vi "PicoScope4000aAdvancedTriggerSettings.vi"(0 "handle in":i16=16384, 5 "error in":errorcluster, 6 "Trigger Conditions":T4={"Channel A"=1, "Channel B"=0, "Channel C"=0, "Channel D"=0, "Channel E"=0, "Channel F"=0, "Channel G"=0, "Channel H"=0, "Ext"=0, "Aux"=0, "PWQ"=0, "Condition Logic"=0} {"Channel H" items=["Don't Care", "True", "False"]; "Channel G" items=["Don't Care", "True", "False"]; "Channel F" items=["Don't Care", "True", "False"]; "Channel E" items=["Don't Care", "True", "False"]; "PWQ" items=["Don't Care", "True", "False"]; "Aux" items=["Don't Care", "True", "False"]; "Ext" items=["Don't Care", "True", "False"]; "Channel D" items=["Don't Care", "True", "False"]; "Channel C" items=["Don't Care", "True", "False"]; "Channel B" items=["Don't Care", "True", "False"]; "Channel A" items=["Don't Care", "True", "False"]; "Condition Logic" items=["AND", "OR", "XOR"]}, 8 "Channel Trigger Properties":T2={"Channel A Trigger Properties"={"thresholdUpper"=0, "thresholdUpperHysteresis"=0, "thresholdLower"=0, "thresholdLowerHysteresis"=0, "Threshold Mode"=0, "Direction"=2, "Available"=TRUE}, "Channel B Trigger Properties"={"thresholdUpper"=0, "thresholdUpperHysteresis"=0, "thresholdLower"=0, "thresholdLowerHysteresis"=0, "Threshold Mode"=0, "Direction"=2, "Available"=FALSE}, "Channel C Trigger Properties"={"thresholdUpper"=0, "thresholdUpperHysteresis"=0, "thresholdLower"=0, "thresholdLowerHysteresis"=0, "Threshold Mode"=0, "Direction"=2, "Available"=FALSE}, "Channel D Trigger Properties"={"thresholdUpper"=0, "thresholdUpperHysteresis"=0, "thresholdLower"=0, "thresholdLowerHysteresis"=0, "Threshold Mode"=0, "Direction"=2, "Available"=FALSE}, "Channel E Trigger Properties"={"thresholdUpper"=0, "thresholdUpperHysteresis"=0, "thresholdLower"=0, "thresholdLowerHysteresis"=0, "Threshold Mode"=0, "Direction"=2, "Available"=FALSE}, "Channel F Trigger Properties"={"thresholdUpper"=0, "thresholdUpperHysteresis"=0, "thresholdLower"=0, "thresholdLowerHysteresis"=0, "Threshold Mode"=0, "Direction"=2, "Available"=FALSE}, "Channel G Trigger Properties"={"thresholdUpper"=0, "thresholdUpperHysteresis"=0, "thresholdLower"=0, "thresholdLowerHysteresis"=0, "Threshold Mode"=0, "Direction"=2, "Available"=FALSE}, "Channel H Trigger Properties"={"thresholdUpper"=0, "thresholdUpperHysteresis"=0, "thresholdLower"=0, "thresholdLowerHysteresis"=0, "Threshold Mode"=0, "Direction"=2, "Available"=FALSE}} {"Channel H Trigger Properties"."Direction" items=["Above / Inside", "Below / Outside", "Rising / Enter", "Falling / Exit", "Rising or Falling / Enter or Exit", "Above Lower", "Below Lower", "Rising Lower", "Falling Lower", "Positive Runt", "Negative Runt"]; "Channel H Trigger Properties"."Threshold Mode" items=["Level", "Window"]; "Channel G Trigger Properties"."Direction" items=["Above / Inside", "Below / Outside", "Rising / Enter", "Falling / Exit", "Rising or Falling / Enter or Exit", "Above Lower", "Below Lower", "Rising Lower", "Falling Lower", "Positive Runt", "Negative Runt"]; "Channel G Trigger Properties"."Threshold Mode" items=["Level", "Window"]; "Channel F Trigger Properties"."Direction" items=["Above / Inside", "Below / Outside", "Rising / Enter", "Falling / Exit", "Rising or Falling / Enter or Exit", "Above Lower", "Below Lower", "Rising Lower", "Falling Lower", "Positive Runt", "Negative Runt"]; "Channel F Trigger Properties"."Threshold Mode" items=["Level", "Window"]; "Channel E Trigger Properties"."Direction" items=["Above / Inside", "Below / Outside", "Rising / Enter", "Falling / Exit", "Rising or Falling / Enter or Exit", "Above Lower", "Below Lower", "Rising Lower", "Falling Lower", "Positive Runt", "Negative Runt"]; "Channel E Trigger Properties"."Threshold Mode" items=["Level", "Window"]; "Channel D Trigger Properties"."Direction" items=["Above / Inside", "Below / Outside", "Rising / Enter", "Falling / Exit", "Rising or Falling / Enter or Exit", "Above Lower", "Below Lower", "Rising Lower", "Falling Lower", "Positive Runt", "Negative Runt"]; "Channel D Trigger Properties"."Threshold Mode" items=["Level", "Window"]; "Channel C Trigger Properties"."Direction" items=["Above / Inside", "Below / Outside", "Rising / Enter", "Falling / Exit", "Rising or Falling / Enter or Exit", "Above Lower", "Below Lower", "Rising Lower", "Falling Lower", "Positive Runt", "Negative Runt"]; "Channel C Trigger Properties"."Threshold Mode" items=["Level", "Window"]; "Channel B Trigger Properties"."Direction" items=["Above / Inside", "Below / Outside", "Rising / Enter", "Falling / Exit", "Rising or Falling / Enter or Exit", "Above Lower", "Below Lower", "Rising Lower", "Falling Lower", "Positive Runt", "Negative Runt"]; "Channel B Trigger Properties"."Threshold Mode" items=["Level", "Window"]; "Channel A Trigger Properties"."Direction" items=["Above / Inside", "Below / Outside", "Rising / Enter", "Falling / Exit", "Rising or Falling / Enter or Exit", "Above Lower", "Below Lower", "Rising Lower", "Falling Lower", "Positive Runt", "Negative Runt"]; "Channel A Trigger Properties"."Threshold Mode" items=["Level", "Window"]}, 9 "Addition Trigger Properties":T3={"Ext. Trigger Properties"={"thresholdUpper"=0, "thresholdUpperHysteresis"=0, "thresholdLower"=0, "thresholdLowerHysteresis"=0, "Threshold Mode"=0, "Direction"=2, "Available"=FALSE}, "Aux. Trigger Properties (DO NOT USE)"={"thresholdUpper"=0, "thresholdUpperHysteresis"=0, "thresholdLower"=0, "thresholdLowerHysteresis"=0, "Threshold Mode"=0, "Direction"=2, "Available"=FALSE}} {"Aux. Trigger Properties (DO NOT USE)"."Direction" items=["Above / Inside", "Below / Outside", "Rising / Enter", "Falling / Exit", "Rising or Falling / Enter or Exit", "Above Lower", "Below Lower", "Rising Lower", "Falling Lower", "Positive Runt", "Negative Runt"]; "Aux. Trigger Properties (DO NOT USE)"."Threshold Mode" items=["Level", "Window"]; "Ext. Trigger Properties"."Direction" items=["Above / Inside", "Below / Outside", "Rising / Enter", "Falling / Exit", "Rising or Falling / Enter or Exit", "Above Lower", "Below Lower", "Rising Lower", "Falling Lower", "Positive Runt", "Negative Runt"]; "Ext. Trigger Properties"."Threshold Mode" items=["Level", "Window"]}, 10 "Auto Trigger (ms)":i32=1000, 11 "Pulse Width Qualifier Conditions":T1 {"Channel H" items=["Don't Care", "True", "False"]; "Channel G" items=["Don't Care", "True", "False"]; "Channel F" items=["Don't Care", "True", "False"]; "Channel E" items=["Don't Care", "True", "False"]; "Aux" items=["Don't Care", "True", "False"]; "Ext" items=["Don't Care", "True", "False"]; "Channel D" items=["Don't Care", "True", "False"]; "Channel C" items=["Don't Care", "True", "False"]; "Channel B" items=["Don't Care", "True", "False"]; "Channel A" items=["Don't Care", "True", "False"]; "Condition Logic" items=["AND", "OR", "XOR"]}, 12 "Trigger Delay":u32, 13 "Pulse Width Qualifier Settings":T5={"Direction"=2, "Lower Limit"=0, "Upper Limit"=0, "Pulse Width Type"=0} {"Pulse Width Type" items=["None", "Less Than", "Greater Than", "In Range", "Out of Range"]; "Direction" items=["Rising"=2, "Falling"=3, "Rising Lower"=7, "Above"=0, "Below"=1, "Rising or Falling"=4, "Falling Lower"=8, "Below Lower"=6, "Above Lower"=5]}) -> (14 "handle out":i16=16384, 19 "error out":errorcluster)   [LabVIEW 2010]
doc: "This VI is an interface for the advanced trigger features of the oscilloscope.\nA simple trigger can be set using PicoScopeXXXXSettings.vi, in which case it is not necessary to use this VI."
uses:
  Program Files/Pico Technology/SDK/lib/ps4000a.dll
panel:
  in  "PWQ Info Action XOR":bool=TRUE
  in  "PWQ Info Action OR":bool=TRUE
  in  "SetTrigger Info Action XOR":bool=TRUE
  out "XOR Debug Array":u32[][](array[numeric])
  in  "SetTrigger Info Action OR":bool=TRUE
  # "For Condition Logic Suggested settings;\nFor AND, XOR logic-(parallel triggers)\nUse level-type triggers (Level or Inside/outside Window Triggers)\n\nFor OR logic- (single channel)\nUse edge types (e.g. rising, falling, entering window)"
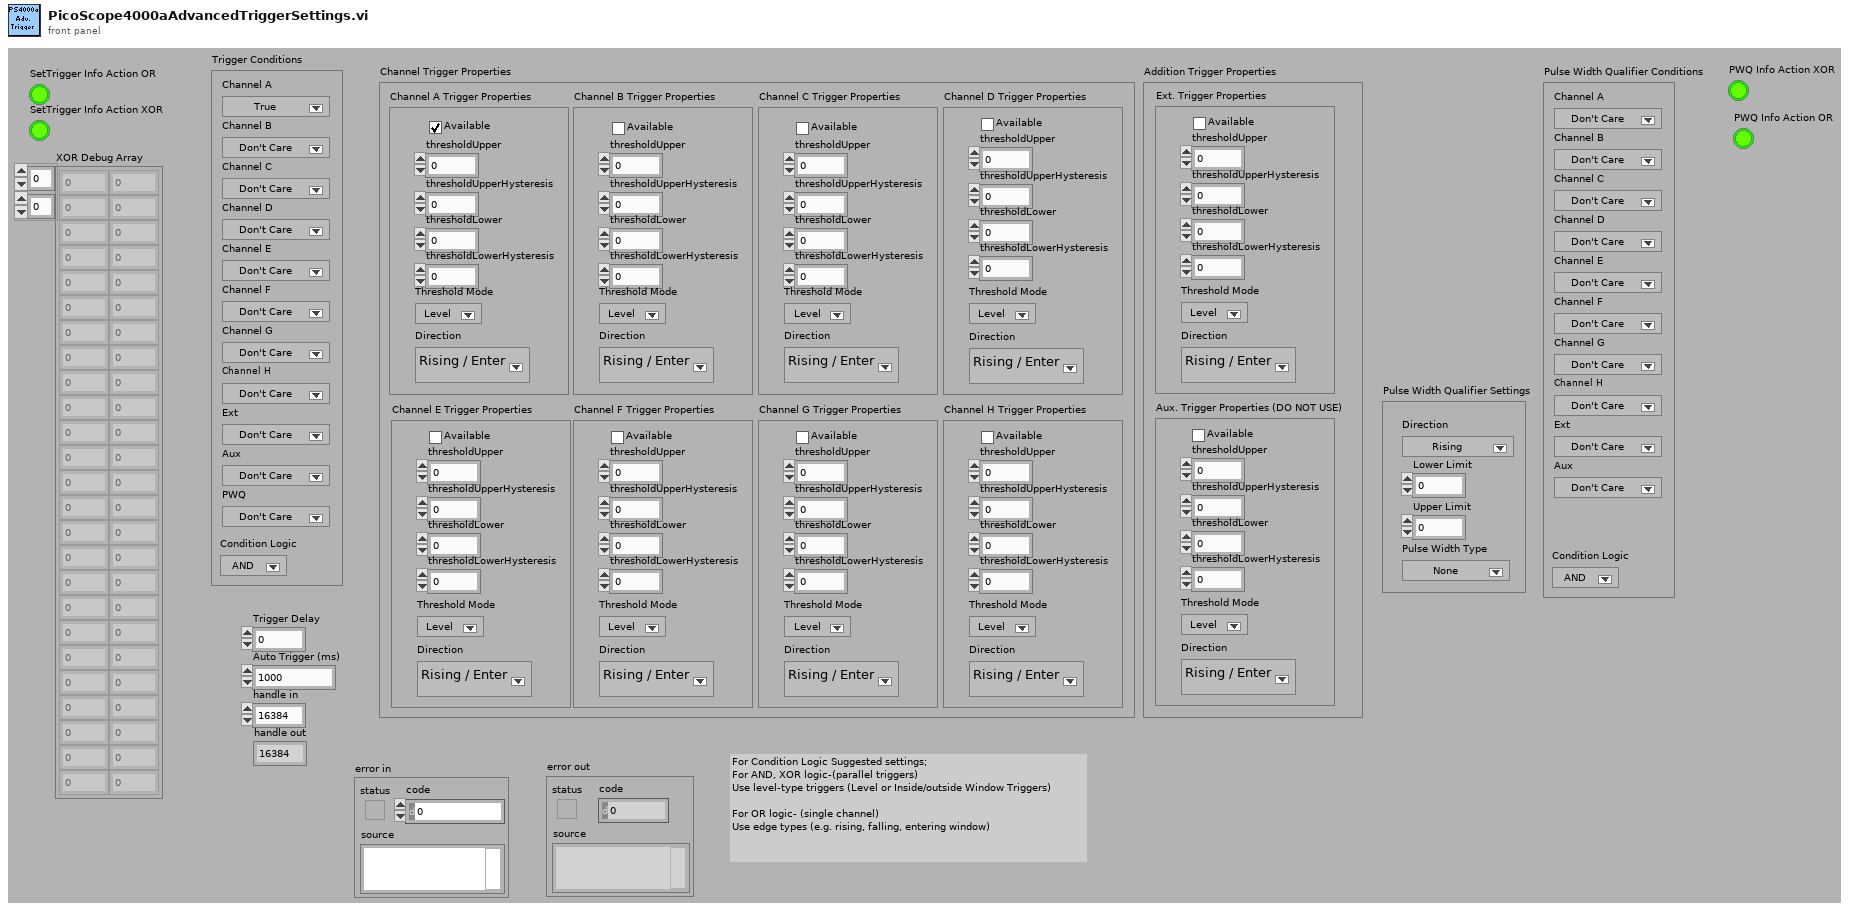
[diagram p1: front panel]
types:
  T1 = cluster{"Channel A":u16, "Channel B":u16, "Channel C":u16, "Channel D":u16, "Channel E":u16, "Channel F":u16, "Channel G":u16, "Channel H":u16, "Ext":u16, "Aux":u16, "Condition Logic":u16}
  T2 = cluster{"Channel A Trigger Properties":cluster{"thresholdUpper":i16, "thresholdUpperHysteresis":u16, "thresholdLower":i16, "thresholdLowerHysteresis":u16, "Threshold Mode":i32, "Direction":i32, "Available":bool}, "Channel B Trigger Properties":cluster{"thresholdUpper":i16, "thresholdUpperHysteresis":u16, "thresholdLower":i16, "thresholdLowerHysteresis":u16, "Threshold Mode":i32, "Direction":i32, "Available":bool}, "Channel C Trigger Properties":cluster{"thresholdUpper":i16, "thresholdUpperHysteresis":u16, "thresholdLower":i16, "thresholdLowerHysteresis":u16, "Threshold Mode":i32, "Direction":i32, "Available":bool}, "Channel D Trigger Properties":cluster{"thresholdUpper":i16, "thresholdUpperHysteresis":u16, "thresholdLower":i16, "thresholdLowerHysteresis":u16, "Threshold Mode":i32, "Direction":i32, "Available":bool}, "Channel E Trigger Properties":cluster{"thresholdUpper":i16, "thresholdUpperHysteresis":u16, "thresholdLower":i16, "thresholdLowerHysteresis":u16, "Threshold Mode":i32, "Direction":i32, "Available":bool}, "Channel F Trigger Properties":cluster{"thresholdUpper":i16, "thresholdUpperHysteresis":u16, "thresholdLower":i16, "thresholdLowerHysteresis":u16, "Threshold Mode":i32, "Direction":i32, "Available":bool}, "Channel G Trigger Properties":cluster{"thresholdUpper":i16, "thresholdUpperHysteresis":u16, "thresholdLower":i16, "thresholdLowerHysteresis":u16, "Threshold Mode":i32, "Direction":i32, "Available":bool}, "Channel H Trigger Properties":cluster{"thresholdUpper":i16, "thresholdUpperHysteresis":u16, "thresholdLower":i16, "thresholdLowerHysteresis":u16, "Threshold Mode":i32, "Direction":i32, "Available":bool}}
  T3 = cluster{"Ext. Trigger Properties":cluster{"thresholdUpper":i16, "thresholdUpperHysteresis":u16, "thresholdLower":i16, "thresholdLowerHysteresis":u16, "Threshold Mode":i32, "Direction":i32, "Available":bool}, "Aux. Trigger Properties (DO NOT USE)":cluster{"thresholdUpper":i16, "thresholdUpperHysteresis":u16, "thresholdLower":i16, "thresholdLowerHysteresis":u16, "Threshold Mode":i32, "Direction":i32, "Available":bool}}
  T4 = cluster{"Channel A":u16, "Channel B":u16, "Channel C":u16, "Channel D":u16, "Channel E":u16, "Channel F":u16, "Channel G":u16, "Channel H":u16, "Ext":u16, "Aux":u16, "PWQ":u16, "Condition Logic":u16}
  T5 = cluster{"Direction":u32, "Lower Limit":u32, "Upper Limit":u32, "Pulse Width Type":u32}
  T6 = cluster{"thresholdUpper":i16, "thresholdUpperHysteresis":u16, "thresholdLower":i16, "thresholdLowerHysteresis":u16, "Threshold Mode":i32, "Direction":i32, "Available":bool}[]
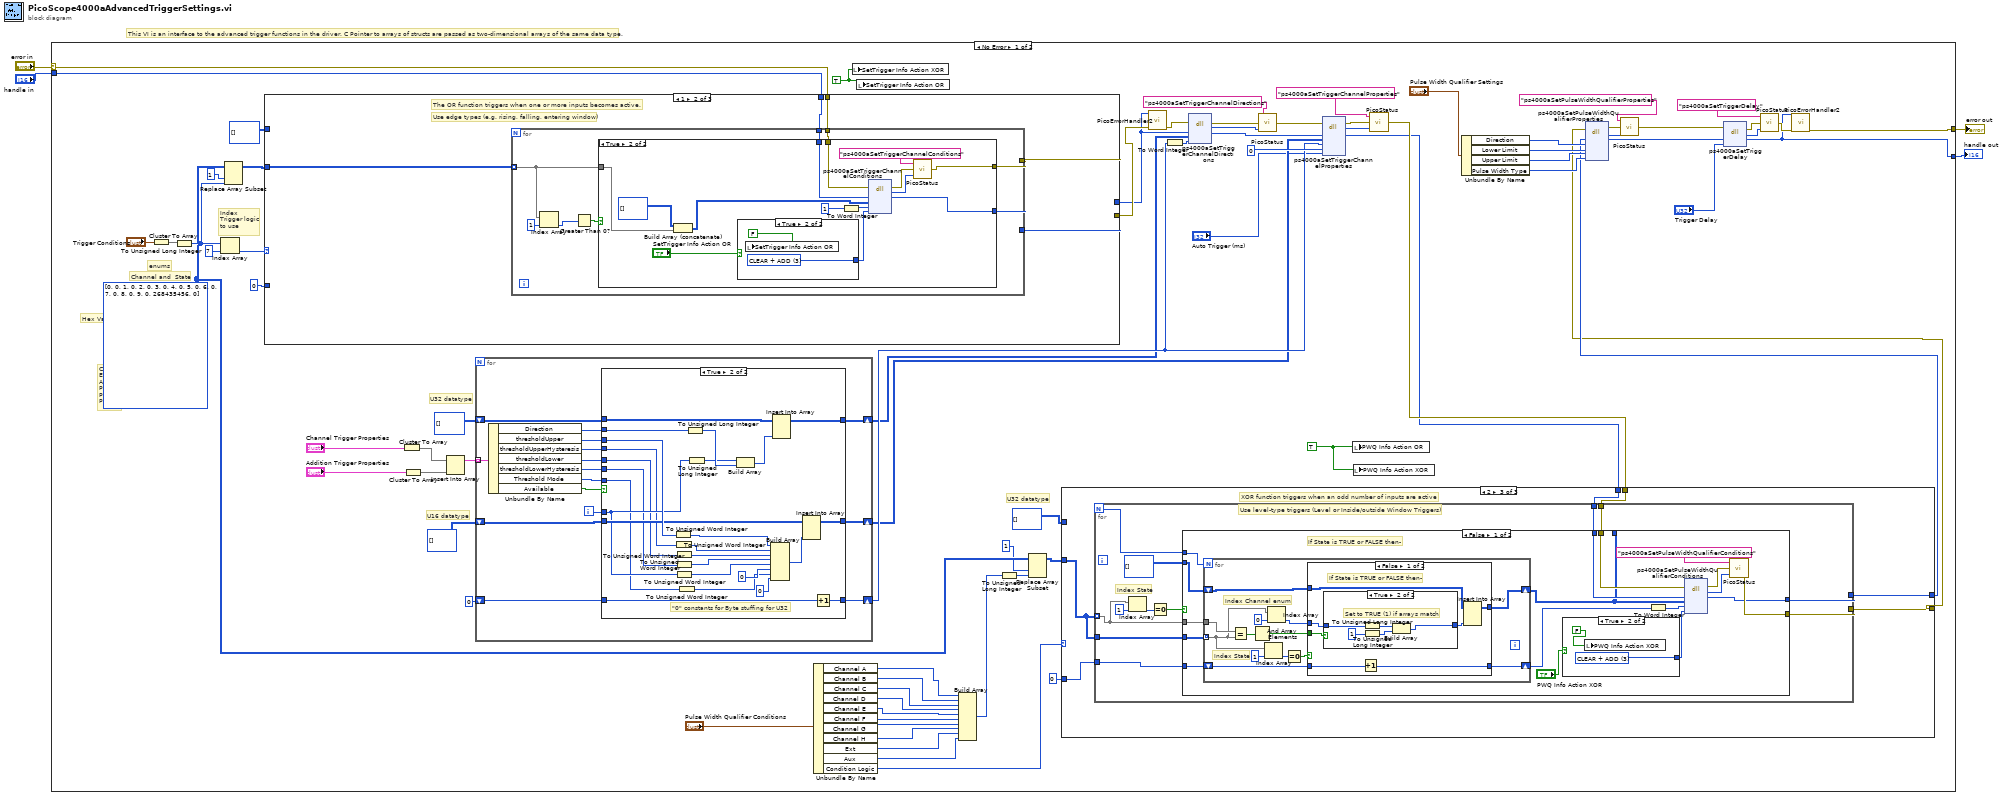
[diagram p0: block diagram]
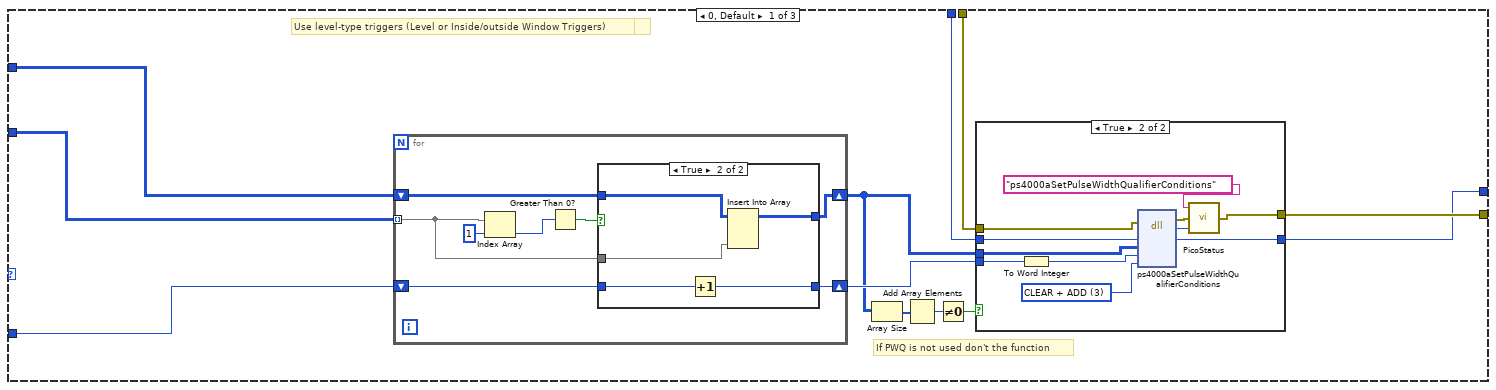
[diagram p2: hidden frame]
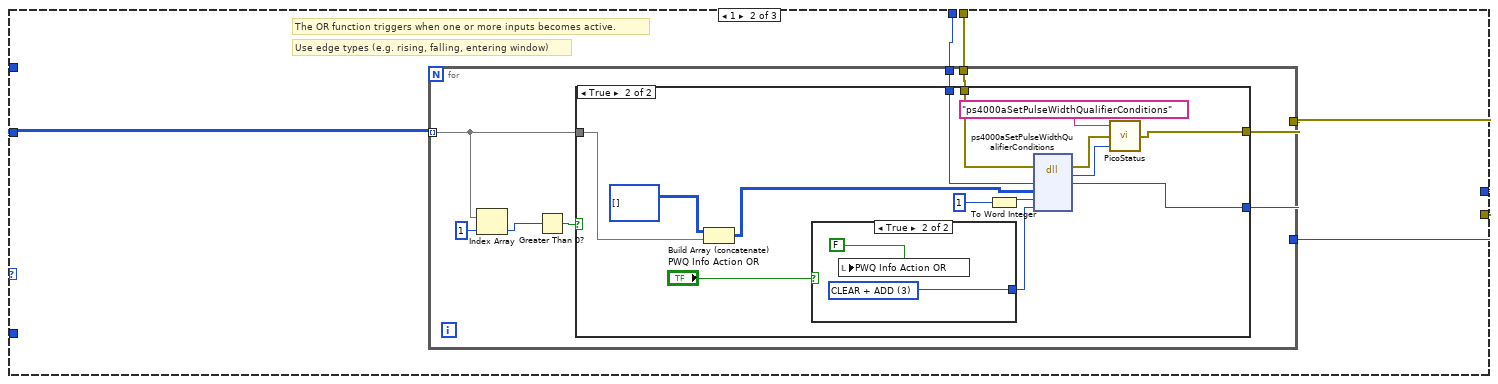
[diagram p5: hidden frame]
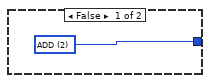
[diagram p7: hidden frame]
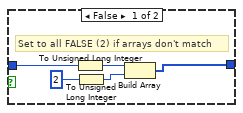
[diagram p8: hidden frame]
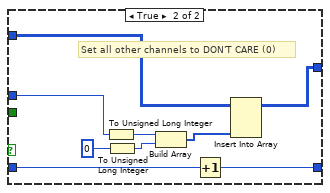
[diagram p9: hidden frame]
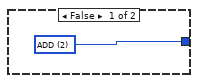
[diagram p10: hidden frame]
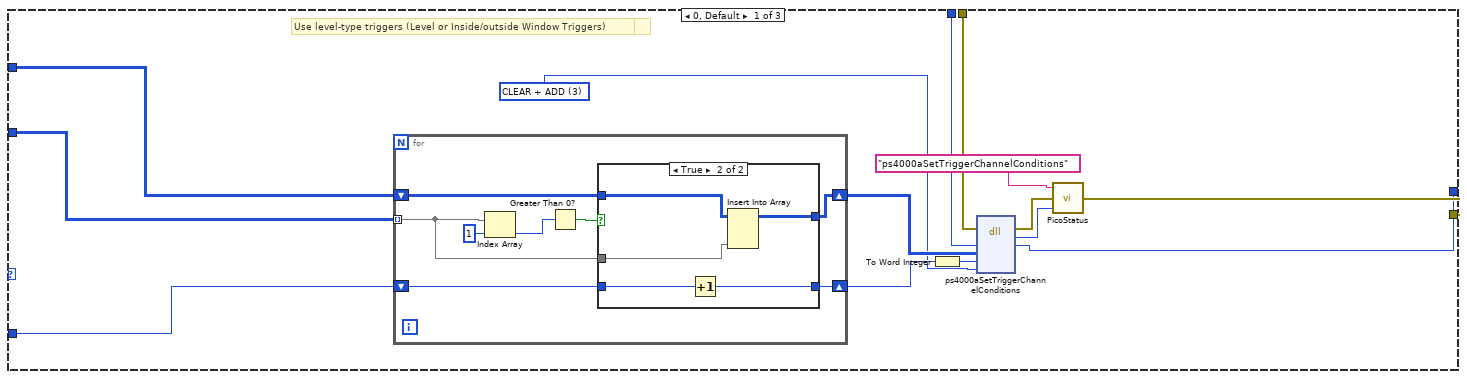
[diagram p12: hidden frame]
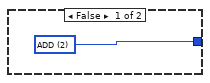
[diagram p15: hidden frame]
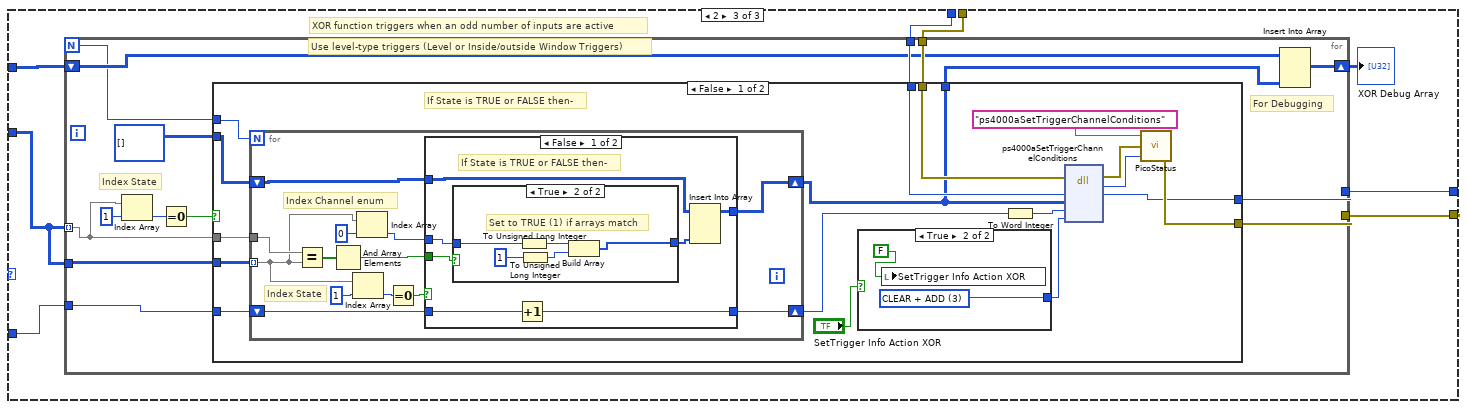
[diagram p16: hidden frame]
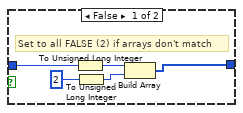
[diagram p17: hidden frame]
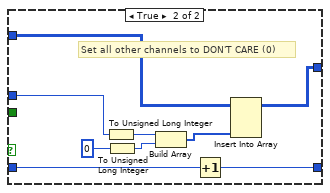
[diagram p18: hidden frame]
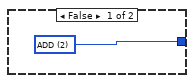
[diagram p19: hidden frame]
diagram:
  # "This VI is an interface to the advanced trigger functions in the driver. C Pointer to arrays of structs are passed as two-dimensional arrays of the same data type."
  n1 = case shown="No Error" "error in" {
    selector: "error in" -> [w36 w424]
    tunnel: "handle in" -> [w35 w425]
    tunnel: [w52 w425] -> w2
    tunnel: [w53 w424] -> w1
    frame No Error {
      w5 = TRUE ("PWQ Info Action XOR")
      w42 = TRUE ("Boolean")
      w20 = u32[][] [[0, 0], [1, 0], [2, 0], [3, 0], [4, 0], [5, 0], [6, 0], [7, 0], [8, 0], [9, 0], [268435456, 0]]
      # "U32 datatype"
      # "Index\nTrigger logic\nto use"
      # "enums"
      # "Ch H\nExt\nAux\nPWQ\nPort0\nPort1"
      # "Channel and  State"
      # "Hex Values"
      # "U16 datatype"
      # "U32 datatype"
      n2 = Cluster To Array(cluster="Trigger Conditions") -> (array=w60:u16[])
      n3 = To Unsigned Long Integer(number=w60) -> (unsigned 32bit integer=w55:u32[])
      n4 = Index Array(array=w55, index=7) -> (element=w41:u32)
      n5 = Replace Array Subset(array=w20, new element=w55, index (col)=1 ("disabled index (col)")) -> (w40:u32[][])  [unwired: 1 in]
      n6 = case shown="1" w41 {
        tunnel: u32[][] [] -> [w248 _ w299]
        tunnel: i16 0 -> [w247 _ w296]
        tunnel: w36 -> [w241 w268 w303]
        tunnel: w35 -> [w240 w267 w302]
        tunnel: [w237 w266 w301] -> w38
        tunnel: [w236 w265 w300] -> w37
        tunnel: w40 -> [w235 w264 w297]
        frame 0, Default {
          w238 = u32 3 items=["CLEAR + ADD"=3, "CLEAR"=1, "ADD"=2] ("Condition Action")
          # "AND function requires both inputs to be active before it will trigger."
          # "Use level-type triggers (Level or Inside/outside Window Triggers)"
          n7 = for {
            shift-right: [w255] -> w243
            shift-left: w247 -> [w254]
            shift-right: [w253] -> w239
            shift-left: w248 -> [w256]
            tunnel: w235 -> [w251] mode=indexing
            n8 = Index Array(array=w251, index=1) -> (element=w250:u32)
            n9 = Greater Than 0?(x=w250) -> (x > 0?=w252:bool)
            n10 = case shown="True" w252 {
              tunnel: w256 -> [w258 w263]
              tunnel: [w258 w262] -> w253
              tunnel: [w257 w261] -> w255
              tunnel: w254 -> [w257 w260]
              tunnel: w251 -> [_ w259]
              frame False {
              }
              frame True {
                n11 = Increment(x=w260) -> (x+1=w261:i16)
                n12 = Insert Into Array(array=w263, new element=w259) -> (w262:u32[][])  [unwired: 2 in]
              }
            }
          }
          n13 = To Word Integer(number=w243) -> (16bit integer=w246:i16)
          n14 = dll-call lib="/Program Files/Pico Technology/SDK/lib/ps4000a.dll" fn="ps4000aSetTriggerChannelConditions" ("ps3000.dll:_ps3000_open_unit@0")(error in=w241, "handle"=w240, "conditions"=w239, "nConditions"=w246, "info"=w238) -> (error out=w245:errorcluster, "PICO_STATUS"=w244:u32, "handle"=w236:i16)  [unwired: 5 in, 1 out]
          n15 = call "PicoStatus.vi"("PICO STATUS"=w244, "error in"=w245, "source"="ps4000aSetTriggerChannelConditions") -> ("error out"=w237:errorcluster)
        }
        frame 1 {
          # "Use edge types (e.g. rising, falling, entering window)"
          # "The OR function triggers when one or more inputs becomes active."
          n16 = for {
            tunnel: w268 -> [w276]
            tunnel: w267 -> [w275]
            tunnel: [w274] -> w266
            tunnel: [w273] -> w265
            tunnel: w264 -> [w271] mode=indexing
            n17 = Index Array(array=w271, index=1) -> (element=w270:u32)
            n18 = Greater Than 0?(x=w270) -> (x > 0?=w269:bool)
            n19 = case shown="True" w269 {
              tunnel: w276 -> [w277 w288]
              tunnel: w275 -> [w278 w287]
              tunnel: [w277 w285] -> w274
              tunnel: [w278 w284] -> w273
              tunnel: w271 -> [_ w279]
              frame False {
              }
              frame True {
                n20 = Build Array (concatenate)(u32[][] [], w279) -> (w281:u32[][])
                n21 = case shown="True" "SetTrigger Info Action OR" {
                  tunnel: [w293 w295] -> w286
                  frame False {
                    w293 = u32 2 items=["CLEAR"=1, "ADD"=2, "CLEAR + ADD"=3] ("Condition Action")
                  }
                  frame True {
                    w295 = u32 3 items=["CLEAR"=1, "ADD"=2, "CLEAR + ADD"=3] ("Condition Action")
                    n22 = local write "SetTrigger Info Action OR"(FALSE ("Boolean")) -> ()
                  }
                }
                n23 = To Word Integer(number=i16 1) -> (16bit integer=w292:i16)
                n24 = dll-call lib="/Program Files/Pico Technology/SDK/lib/ps4000a.dll" fn="ps4000aSetTriggerChannelConditions" ("ps3000.dll:_ps3000_open_unit@0")(error in=w288, "handle"=w287, "conditions"=w281, "nConditions"=w292, "info"=w286) -> (error out=w291:errorcluster, "PICO_STATUS"=w290:u32, "handle"=w284:i16)  [unwired: 5 in, 1 out]
                n25 = call "PicoStatus.vi"("PICO STATUS"=w290, "error in"=w291, "source"="ps4000aSetTriggerChannelConditions") -> ("error out"=w285:errorcluster)
              }
            }
          }
        }
        frame 2 {
          # "Use level-type triggers (Level or Inside/outside Window Triggers)"
          # "XOR function triggers when an odd number of inputs are active"
          n26 = for {
            N -> [w311]
            tunnel: w303 -> [w318]
            tunnel: w302 -> [w317]
            tunnel: [w316] -> w301
            tunnel: [w315] -> w300
            shift-right: [w313] -> w298
            shift-left: w299 -> [w314]
            tunnel: w297 -> [w305] mode=indexing
            tunnel: w297 -> [w308]
            tunnel: w296 -> [w309]
            # "Index State"
            # "For Debugging"
            n27 = Index Array(array=w305, index=1) -> (element=w306:u32)
            n28 = Equal To 0?(x=w306) -> (x = 0?=w304:bool)
            n29 = case shown="False" w304 {
              tunnel: w318 -> [w335 w378]
              tunnel: w317 -> [w334 w379]
              tunnel: [w333 w378] -> w316
              tunnel: [w332 w379] -> w315
              tunnel: [w330 w380] -> w312
              tunnel: w311 -> [w329 _]
              tunnel: u32[][] [] -> [w328 w380]
              tunnel: w309 -> [w327 _]
              tunnel: w308 -> [w326 _]
              tunnel: w305 -> [w325 _]
              frame False {
                # "If State is TRUE or FALSE then-"
                n30 = for {
                  N: w329 -> [_]
                  shift-right: [w347] -> w331
                  shift-left: w327 -> [w348]
                  shift-right: [w336] -> w330
                  shift-left: w328 -> [w337]
                  tunnel: w325 -> [w344]
                  tunnel: w326 -> [w340] mode=indexing
                  # "Index State"
                  # "Index Channel enum"
                  n31 = Equal?(x=w344, y=w340) -> (x = y?=w338:bool[])
                  n32 = And Array Elements(Boolean array=w338) -> (logical AND=w343:bool)
                  n33 = Index Array(array=w340, index=1) -> (element=w341:u32)
                  n34 = Index Array(array=w340, index=0) -> (element=w345:u32)
                  n35 = Equal To 0?(x=w341) -> (x = 0?=w339:bool)
                  n36 = case shown="False" w339 {
                    tunnel: w348 -> [w355 w366]
                    tunnel: [w354 w367] -> w347
                    tunnel: w345 -> [w353 w370]
                    tunnel: w343 -> [w352 _]
                    tunnel: w337 -> [w351 w369]
                    tunnel: [w349 w368] -> w336
                    frame False {
                      # "If State is TRUE or FALSE then-"
                      n37 = case shown="True" w352 {
                        tunnel: [w360 w365] -> w350
                        tunnel: w353 -> [w359 w364]
                        frame False {
                          # "Set to all FALSE (2) if arrays don't match"
                          n38 = To Unsigned Long Integer(number=w359) -> (unsigned 32bit integer=w357:u32)
                          n39 = To Unsigned Long Integer(number=u32 2) -> (unsigned 32bit integer=w358:u32)
                          n40 = Build Array(w357, w358) -> (w360:u32[])
                        }
                        frame True {
                          # "Set to TRUE (1) if arrays match"
                          n41 = To Unsigned Long Integer(number=w364) -> (unsigned 32bit integer=w362:u32)
                          n42 = To Unsigned Long Integer(number=u32 1) -> (unsigned 32bit integer=w363:u32)
                          n43 = Build Array(w362, w363) -> (w365:u32[])
                        }
                      }
                      n44 = Increment(x=w355) -> (x+1=w354:i16)
                      n45 = Insert Into Array(array=w351, new element=w350) -> (w349:u32[][])  [unwired: 2 in]
                    }
                    frame True {
                      # "Set all other channels to DON'T CARE (0)"
                      n46 = To Unsigned Long Integer(number=w370) -> (unsigned 32bit integer=w372:u32)
                      n47 = To Unsigned Long Integer(number=u32 0) -> (unsigned 32bit integer=w373:u32)
                      n48 = Build Array(w372, w373) -> (w374:u32[])
                      n49 = Increment(x=w366) -> (x+1=w367:i16)
                      n50 = Insert Into Array(array=w369, new element=w374) -> (w368:u32[][])  [unwired: 2 in]
                    }
                  }
                }
                n51 = case shown="True" "SetTrigger Info Action XOR" {
                  tunnel: [w375 w377] -> w319
                  frame False {
                    w375 = u32 2 items=["CLEAR + ADD"=3, "CLEAR"=1, "ADD"=2] ("Condition Action")
                  }
                  frame True {
                    w377 = u32 3 items=["CLEAR + ADD"=3, "CLEAR"=1, "ADD"=2] ("Condition Action")
                    n52 = local write "SetTrigger Info Action XOR"(FALSE ("Boolean")) -> ()
                  }
                }
                n53 = To Word Integer(number=w331) -> (16bit integer=w324:i16)
                n54 = dll-call lib="/Program Files/Pico Technology/SDK/lib/ps4000a.dll" fn="ps4000aSetTriggerChannelConditions" ("ps3000.dll:_ps3000_open_unit@0")(error in=w335, "handle"=w334, "conditions"=w330, "nConditions"=w324, "info"=w319) -> (error out=w323:errorcluster, "PICO_STATUS"=w322:u32, "handle"=w332:i16)  [unwired: 5 in, 1 out]
                n55 = call "PicoStatus.vi"("PICO STATUS"=w322, "error in"=w323, "source"="ps4000aSetTriggerChannelConditions") -> ("error out"=w333:errorcluster)
              }
              frame True {
              }
            }
            n56 = Insert Into Array(array=w314, new element=w312) -> (w313:u32[][])  [unwired: 2 in]
          }
          "XOR Debug Array" <- w298
        }
      }
      n57 = Cluster To Array(cluster="Channel Trigger Properties") -> (array=w30:T6)
      n58 = Cluster To Array(cluster="Addition Trigger Properties") -> (array=w28:T6)
      n59 = Insert Into Array(array=w30, new element=w28) -> (w29:T6)  [unwired: 1 in]
      n60 = for {
        tunnel: w29 -> [w381] mode=indexing
        shift-right: [w388] -> w63
        shift-left: i16 0 -> [w387]
        shift-right: [w385] -> w57
        shift-left: u16[][] [] -> [w386]
        shift-right: [w384] -> w58
        shift-left: u32[][] [] -> [w383]
        i -> [w389]
        n61 = Unbundle By Name(w381) -> ("Direction"=w382:i32, "thresholdUpper"=w395:i16, "thresholdUpperHysteresis"=w394:u16, "thresholdLower"=w393:i16, "thresholdLowerHysteresis"=w392:u16, "Threshold Mode"=w391:i32, "Available"=w390:bool)
        n62 = case shown="True" w390 {
          tunnel: w395 -> [_ w423]
          tunnel: w394 -> [_ w405]
          tunnel: w393 -> [_ w404]
          tunnel: w392 -> [_ w403]
          tunnel: w391 -> [_ w399]
          tunnel: w389 -> [_ w413]
          tunnel: [w398 w421] -> w388
          tunnel: w387 -> [w398 w420]
          tunnel: [w397 w418] -> w385
          tunnel: w386 -> [w397 w417]
          tunnel: [w396 w416] -> w384
          tunnel: w383 -> [w396 w415]
          tunnel: w382 -> [_ w412]
          frame False {
          }
          frame True {
            # "\"0\" constants for Byte stuffing for U32"
            n63 = To Unsigned Word Integer(number=w423) -> (unsigned 16bit integer=w407:u16)
            n64 = To Unsigned Word Integer(number=w405) -> (unsigned 16bit integer=w406:u16)
            n65 = To Unsigned Word Integer(number=w404) -> (unsigned 16bit integer=w402:u16)
            n66 = To Unsigned Word Integer(number=w403) -> (unsigned 16bit integer=w408:u16)
            n67 = To Unsigned Word Integer(number=w413) -> (unsigned 16bit integer=w409:u16)
            n68 = To Unsigned Word Integer(number=w399) -> (unsigned 16bit integer=w400:u16)
            n69 = To Unsigned Long Integer(number=w412) -> (unsigned 32bit integer=w411:u32)
            n70 = To Unsigned Long Integer(number=w413) -> (unsigned 32bit integer=w410:u32)
            n71 = Build Array(w410, w411) -> (w414:u32[])
            n72 = Build Array(w407, w406, w402, w408, w409, u16 0 ("element"), w400, u16 0 ("element")) -> (w419:u16[])
            n73 = Insert Into Array(array=w415, new element=w414) -> (w416:u32[][])  [unwired: 2 in]
            n74 = Insert Into Array(array=w417, new element=w419) -> (w418:u16[][])  [unwired: 2 in]
            n75 = Increment(x=w420) -> (x+1=w421:i16)
          }
        }
      }
      n76 = Unbundle By Name("Pulse Width Qualifier Conditions") -> ("Channel A"=w15:u16, "Channel B"=w14:u16, "Channel C"=w13:u16, "Channel D"=w12:u16, "Channel E"=w11:u16, "Channel F"=w10:u16, "Channel G"=w9:u16, "Channel H"=w8:u16, "Ext"=w7:u16, "Aux"=w6:u16, "Condition Logic"=w27:u16)
      n77 = local write "SetTrigger Info Action XOR"(w42) -> ()
      n78 = local write "SetTrigger Info Action OR"(w42) -> ()
      n79 = Build Array(w15, w14, w13, w12, w11, w10, w9, w8, w7, w6) -> (w56:u16[])
      n80 = To Unsigned Long Integer(number=w56) -> (unsigned 32bit integer=w19:u32[])
      n81 = Replace Array Subset(array=w20, new element=w19, index (col)=1 ("disabled index (col)")) -> (w18:u32[][])  [unwired: 1 in]
      n82 = call "PicoErrorHandler2.vi"("error in (no error)"=w38, "handle In"=w37) -> ("error out"=w44:errorcluster)  [unwired: 9 in]
      n83 = To Word Integer(number=w63) -> (16bit integer=w64:i16)
      n84 = dll-call lib="/Program Files/Pico Technology/SDK/lib/ps4000a.dll" fn="ps4000aSetTriggerChannelDirections" ("ps3000.dll:_ps3000_open_unit@0")(error in=w44, "handle"=w37, "directions"=w58, "nDirections"=w64) -> (error out=w78:errorcluster, "PICO_STATUS"=w79:u32, "handle"=w81:i16)  [unwired: 4 in, 1 out]
      n85 = call "PicoStatus.vi"("PICO STATUS"=w79, "error in"=w78, "source"="ps4000aSetTriggerChannelDirections") -> ("error out"=w72:errorcluster)
      n86 = dll-call lib="/Program Files/Pico Technology/SDK/lib/ps4000a.dll" fn="ps4000aSetTriggerChannelProperties" ("ps3000.dll:_ps3000_open_unit@0")(error in=w72, "handle"=w81, "channelProperties"=w57, "nChannelProperties"=w63, "auxOutputEnable"=i16 0, "autoTriggerMilliseconds"="Auto Trigger (ms)") -> (error out=w76:errorcluster, "PICO_STATUS"=w77:u32, "handle"=w23:i16)  [unwired: 6 in, 1 out]
      n87 = local write "PWQ Info Action OR"(w5) -> ()
      n88 = local write "PWQ Info Action XOR"(w5) -> ()
      n89 = call "PicoStatus.vi"("PICO STATUS"=w77, "error in"=w76, "source"="ps4000aSetTriggerChannelProperties") -> ("error out"=w24:errorcluster)
      n90 = case shown="2" w27 {
        tunnel: u32[][] [] -> [w94 _ _]
        tunnel: i16 0 -> [w93 _ w155]
        tunnel: w24 -> [w90 w127 w160]
        tunnel: w23 -> [w89 w126 w159]
        tunnel: [w88 w125 w158] -> w21
        tunnel: [w87 w124 w157] -> w22
        tunnel: w18 -> [w91 w123 w156]
        frame 0, Default {
          # "If PWQ is not used don't the function"
          # "AND function requires both inputs to be active before it will trigger."
          # "Use level-type triggers (Level or Inside/outside Window Triggers)"
          n91 = for {
            shift-right: [w114] -> w92
            shift-left: w93 -> [w113]
            shift-right: [w112] -> w86
            shift-left: w94 -> [w115]
            tunnel: w91 -> [w110] mode=indexing
            n92 = Index Array(array=w110, index=1) -> (element=w109:u32)
            n93 = Greater Than 0?(x=w109) -> (x > 0?=w111:bool)
            n94 = case shown="True" w111 {
              tunnel: w115 -> [w117 w122]
              tunnel: [w117 w121] -> w112
              tunnel: [w116 w120] -> w114
              tunnel: w113 -> [w116 w119]
              tunnel: w110 -> [_ w118]
              frame False {
              }
              frame True {
                n95 = Increment(x=w119) -> (x+1=w120:i16)
                n96 = Insert Into Array(array=w122, new element=w118) -> (w121:u32[][])  [unwired: 2 in]
              }
            }
          }
          n97 = Array Size(array=w86) -> (size(s)=w84:i32[])
          n98 = Add Array Elements(numeric array=w84) -> (sum=w85:i32)
          n99 = Not Equal To 0?(x=w85) -> (x != 0?=w83:bool)
          n100 = case shown="True" w83 {
            tunnel: w92 -> [_ w107]
            tunnel: w90 -> [w96 w103]
            tunnel: w89 -> [w95 w102]
            tunnel: w86 -> [_ w99]
            tunnel: [w96 w98] -> w88
            tunnel: [w95 w97] -> w87
            frame False {
            }
            frame True {
              w101 = u32 3 items=["CLEAR + ADD"=3, "CLEAR"=1, "ADD"=2] ("Condition Action")
              n101 = To Word Integer(number=w107) -> (16bit integer=w100:i16)
              n102 = dll-call lib="/Program Files/Pico Technology/SDK/lib/ps4000a.dll" fn="ps4000aSetPulseWidthQualifierConditions" ("ps3000.dll:_ps3000_open_unit@0")(error in=w103, "handle"=w102, "conditions"=w99, "nConditions"=w100, "info"=w101) -> (error out=w106:errorcluster, "PICO_STATUS"=w105:u32, "handle"=w97:i16)  [unwired: 5 in, 1 out]
              n103 = call "PicoStatus.vi"("PICO STATUS"=w105, "error in"=w106, "source"="ps4000aSetPulseWidthQualifierConditions") -> ("error out"=w98:errorcluster)
            }
          }
        }
        frame 1 {
          # "Use edge types (e.g. rising, falling, entering window)"
          # "The OR function triggers when one or more inputs becomes active."
          n104 = for {
            tunnel: w127 -> [w135]
            tunnel: w126 -> [w134]
            tunnel: [w133] -> w125
            tunnel: [w132] -> w124
            tunnel: w123 -> [w130] mode=indexing
            n105 = Index Array(array=w130, index=1) -> (element=w129:u32)
            n106 = Greater Than 0?(x=w129) -> (x > 0?=w128:bool)
            n107 = case shown="True" w128 {
              tunnel: w135 -> [w136 w147]
              tunnel: w134 -> [w137 w146]
              tunnel: [w136 w144] -> w133
              tunnel: [w137 w143] -> w132
              tunnel: w130 -> [_ w138]
              frame False {
              }
              frame True {
                n108 = Build Array (concatenate)(u32[][] [], w138) -> (w140:u32[][])
                n109 = case shown="True" "PWQ Info Action OR" {
                  tunnel: [w152 w154] -> w145
                  frame False {
                    w152 = u32 2 items=["CLEAR"=1, "ADD"=2, "CLEAR + ADD"=3] ("Condition Action")
                  }
                  frame True {
                    w154 = u32 3 items=["CLEAR"=1, "ADD"=2, "CLEAR + ADD"=3] ("Condition Action")
                    n110 = local write "PWQ Info Action OR"(FALSE ("Boolean")) -> ()
                  }
                }
                n111 = To Word Integer(number=i16 1) -> (16bit integer=w151:i16)
                n112 = dll-call lib="/Program Files/Pico Technology/SDK/lib/ps4000a.dll" fn="ps4000aSetPulseWidthQualifierConditions" ("ps3000.dll:_ps3000_open_unit@0")(error in=w147, "handle"=w146, "conditions"=w140, "nConditions"=w151, "info"=w145) -> (error out=w150:errorcluster, "PICO_STATUS"=w149:u32, "handle"=w143:i16)  [unwired: 5 in, 1 out]
                n113 = call "PicoStatus.vi"("PICO STATUS"=w149, "error in"=w150, "source"="ps4000aSetPulseWidthQualifierConditions") -> ("error out"=w144:errorcluster)
              }
            }
          }
        }
        frame 2 {
          # "Use level-type triggers (Level or Inside/outside Window Triggers)"
          # "XOR function triggers when an odd number of inputs are active"
          n114 = for {
            N -> [w168]
            tunnel: w160 -> [w172]
            tunnel: w159 -> [w171]
            tunnel: [w170] -> w158
            tunnel: [w169] -> w157
            tunnel: w156 -> [w162] mode=indexing
            tunnel: w156 -> [w165]
            tunnel: w155 -> [w166]
            # "Index State"
            n115 = Index Array(array=w162, index=1) -> (element=w163:u32)
            n116 = Equal To 0?(x=w163) -> (x = 0?=w161:bool)
            n117 = case shown="False" w161 {
              tunnel: w172 -> [w189 w232]
              tunnel: w171 -> [w188 w233]
              tunnel: [w187 w232] -> w170
              tunnel: [w186 w233] -> w169
              tunnel: [w184 w234] -> _
              tunnel: w168 -> [w183 _]
              tunnel: u32[][] [] -> [w182 w234]
              tunnel: w166 -> [w181 _]
              tunnel: w165 -> [w180 _]
              tunnel: w162 -> [w179 _]
              frame False {
                # "If State is TRUE or FALSE then-"
                n118 = for {
                  N: w183 -> [_]
                  shift-right: [w201] -> w185
                  shift-left: w181 -> [w202]
                  shift-right: [w190] -> w184
                  shift-left: w182 -> [w191]
                  tunnel: w179 -> [w198]
                  tunnel: w180 -> [w194] mode=indexing
                  # "Index State"
                  # "Index Channel enum"
                  n119 = Equal?(x=w198, y=w194) -> (x = y?=w192:bool[])
                  n120 = And Array Elements(Boolean array=w192) -> (logical AND=w197:bool)
                  n121 = Index Array(array=w194, index=1) -> (element=w195:u32)
                  n122 = Index Array(array=w194, index=0) -> (element=w199:u32)
                  n123 = Equal To 0?(x=w195) -> (x = 0?=w193:bool)
                  n124 = case shown="False" w193 {
                    tunnel: w202 -> [w209 w220]
                    tunnel: [w208 w221] -> w201
                    tunnel: w199 -> [w207 w224]
                    tunnel: w197 -> [w206 _]
                    tunnel: w191 -> [w205 w223]
                    tunnel: [w203 w222] -> w190
                    frame False {
                      # "If State is TRUE or FALSE then-"
                      n125 = case shown="True" w206 {
                        tunnel: [w214 w219] -> w204
                        tunnel: w207 -> [w213 w218]
                        frame False {
                          # "Set to all FALSE (2) if arrays don't match"
                          n126 = To Unsigned Long Integer(number=w213) -> (unsigned 32bit integer=w211:u32)
                          n127 = To Unsigned Long Integer(number=u32 2) -> (unsigned 32bit integer=w212:u32)
                          n128 = Build Array(w211, w212) -> (w214:u32[])
                        }
                        frame True {
                          # "Set to TRUE (1) if arrays match"
                          n129 = To Unsigned Long Integer(number=w218) -> (unsigned 32bit integer=w216:u32)
                          n130 = To Unsigned Long Integer(number=u32 1) -> (unsigned 32bit integer=w217:u32)
                          n131 = Build Array(w216, w217) -> (w219:u32[])
                        }
                      }
                      n132 = Increment(x=w209) -> (x+1=w208:i16)
                      n133 = Insert Into Array(array=w205, new element=w204) -> (w203:u32[][])  [unwired: 2 in]
                    }
                    frame True {
                      # "Set all other channels to DON'T CARE (0)"
                      n134 = To Unsigned Long Integer(number=w224) -> (unsigned 32bit integer=w226:u32)
                      n135 = To Unsigned Long Integer(number=u32 0) -> (unsigned 32bit integer=w227:u32)
                      n136 = Build Array(w226, w227) -> (w228:u32[])
                      n137 = Increment(x=w220) -> (x+1=w221:i16)
                      n138 = Insert Into Array(array=w223, new element=w228) -> (w222:u32[][])  [unwired: 2 in]
                    }
                  }
                }
                n139 = case shown="True" "PWQ Info Action XOR" {
                  tunnel: [w229 w231] -> w173
                  frame False {
                    w229 = u32 2 items=["CLEAR + ADD"=3, "CLEAR"=1, "ADD"=2] ("Condition Action")
                  }
                  frame True {
                    w231 = u32 3 items=["CLEAR + ADD"=3, "CLEAR"=1, "ADD"=2] ("Condition Action")
                    n140 = local write "PWQ Info Action XOR"(FALSE ("Boolean")) -> ()
                  }
                }
                n141 = To Word Integer(number=w185) -> (16bit integer=w178:i16)
                n142 = dll-call lib="/Program Files/Pico Technology/SDK/lib/ps4000a.dll" fn="ps4000aSetPulseWidthQualifierConditions" ("ps3000.dll:_ps3000_open_unit@0")(error in=w189, "handle"=w188, "conditions"=w184, "nConditions"=w178, "info"=w173) -> (error out=w177:errorcluster, "PICO_STATUS"=w176:u32, "handle"=w186:i16)  [unwired: 5 in, 1 out]
                n143 = call "PicoStatus.vi"("PICO STATUS"=w176, "error in"=w177, "source"="ps4000aSetPulseWidthQualifierConditions") -> ("error out"=w187:errorcluster)
              }
              frame True {
              }
            }
          }
        }
      }
      n144 = Unbundle By Name("Pulse Width Qualifier Settings") -> ("Direction"=w48:u32, "Lower Limit"=w47:u32, "Upper Limit"=w46:u32, "Pulse Width Type"=w45:u32)
      n145 = dll-call lib="/Program Files/Pico Technology/SDK/lib/ps4000a.dll" fn="ps4000aSetPulseWidthQualifierProperties" ("ps3000.dll:_ps3000_open_unit@0")(error in=w21, "handle"=w22, "direction"=w48, "lower"=w47, "upper"=w46, "type"=w45) -> (error out=w51:errorcluster, "PICO_STATUS"=w34:u32, "handle"=w33:i16)  [unwired: 6 in, 1 out]
      n146 = call "PicoStatus.vi"("PICO STATUS"=w34, "error in"=w51, "source"="ps4000aSetPulseWidthQualifierProperties") -> ("error out"=w49:errorcluster)
      n147 = dll-call lib="/Program Files/Pico Technology/SDK/lib/ps4000a.dll" fn="ps4000aSetTriggerDelay" ("ps3000.dll:_ps3000_open_unit@0")(error in=w49, "handle"=w33, "delay"="Trigger Delay") -> (error out=w74:errorcluster, "PICO_STATUS"=w75:u32, "handle"=w52:i16)  [unwired: 3 in, 1 out]
      n148 = call "PicoStatus.vi"("PICO STATUS"=w75, "error in"=w74, "source"="ps4000aSetTriggerDelay") -> ("error out"=w73:errorcluster)
      n149 = call "PicoErrorHandler2.vi"("error in (no error)"=w73, "handle In"=w52) -> ("error out"=w53:errorcluster)  [unwired: 9 in]
    }
    frame Error {
    }
  }
  "handle out" <- w2
  "error out" <- w1
